vi "fail quit test.vi"(10 "EN":bool, 11 "数组":bool[](array[boolean])) -> (3 "布尔":bool)   [LabVIEW 2018]
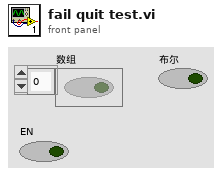
[diagram p1: front panel]
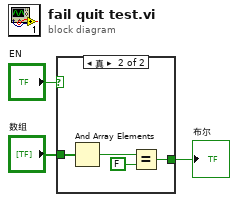
[diagram p0: block diagram]
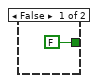
[diagram p2: hidden frame]
diagram:
  n1 = case shown="真" "EN" {
    tunnel: "数组" -> [_ w6]
    tunnel: [FALSE w5] -> w2
    frame False {
    }
    frame True {
      n2 = And Array Elements(Boolean array=w6) -> (logical AND=w8:bool)
      n3 = Equal?(x=w8, y=FALSE) -> (x = y?=w5:bool)
    }
  }
  "布尔" <- w2
